vi "post_dust_event.vi"(8 "error in (no error)":errorcluster, 10 "Signal Array":T1[](array[typedef]), 11 "Cluster":T4 {"File Location" items=["Unknown"=-5, "IDL Processing"=-4, "Writing from Queue"=-3, "Labview Files"=-2, "Retry Labview files"=-1, "Local Cache "=0, "Storage"=1]}) -> (0 "error out":errorcluster, 1 "Experiment Settings":i32, 2 "Dust Event ID":i32, 3 "Test Server":bool)   [LabVIEW 2013]
uses:
  Public API/Post_Dust_Event.ctl
  Controls/File_location.ctl
  Public API/Signal.ctl
  Controls/Role ID.ctl
  Controls/Hardware ID.ctl
  <vilib>/addons/database/Auxilliary.llb/DB Tools Cursor Type.ctl
  <vilib>/addons/database/Connection.llb/Conn Execute.vi
  <vilib>/addons/database/Recordset.llb/Rec Fetch Recordset Data (R).vi
  <vilib>/addons/database/Recordset.llb/Rec Destroy - Connection.vi
  <vilib>/addons/database/_DB Variant To Data/Database Variant To Data.xnode
  <vilib>/addons/database/NI_Database_API.lvlib
panel:
  # "Signal"
  # "Dust Event"
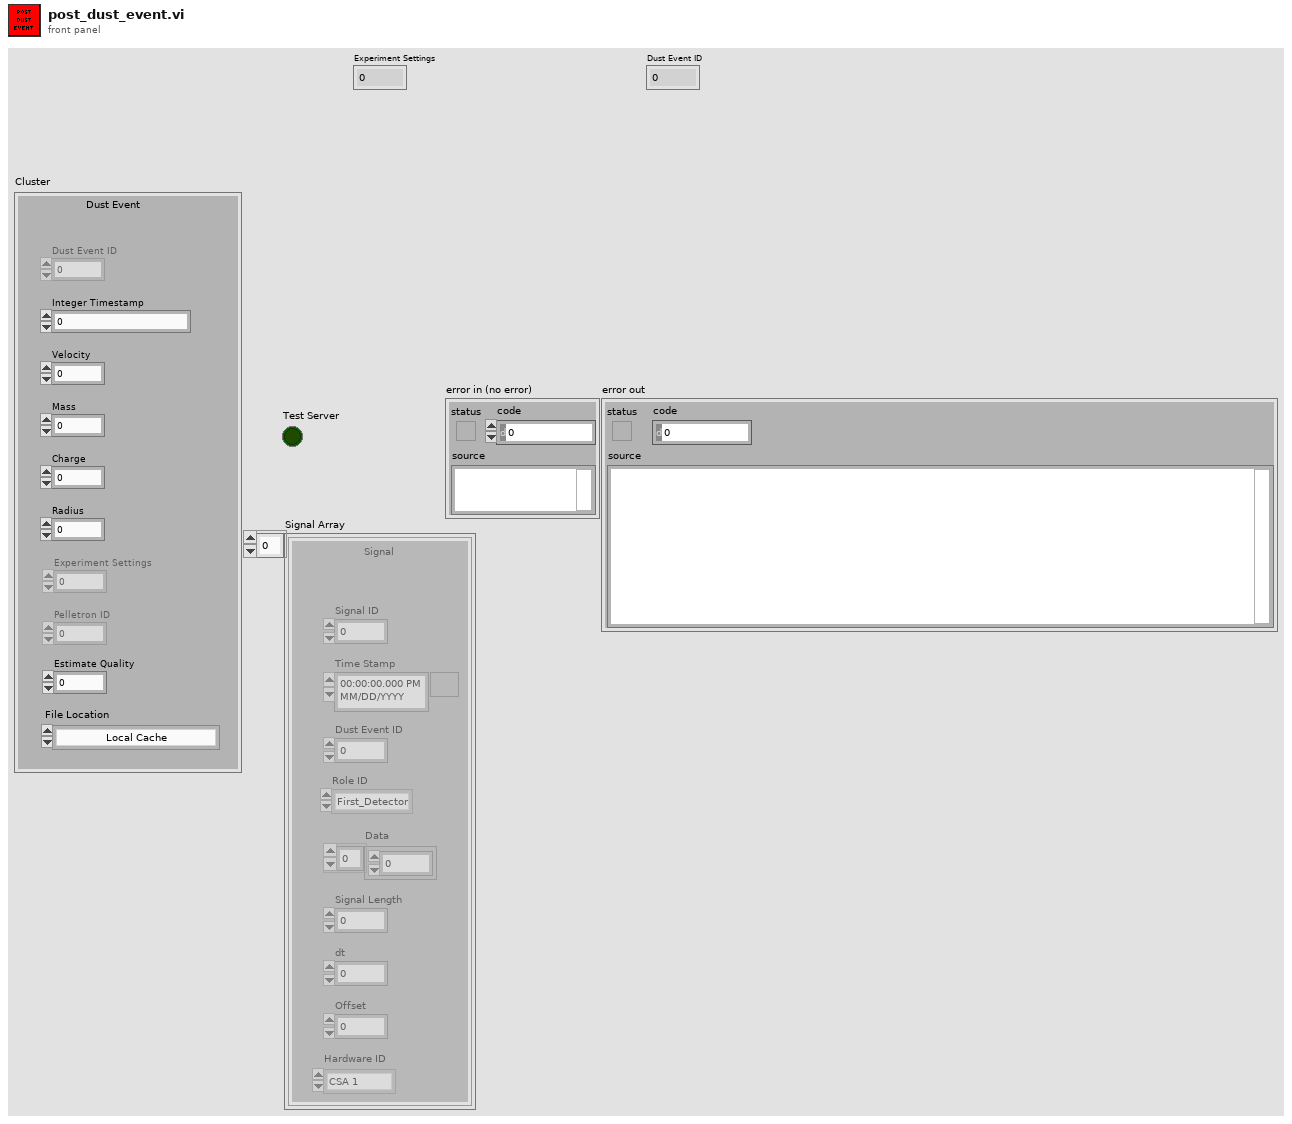
[diagram p1: front panel]
types:
  T1 = typedef "Signal.ctl" = cluster{"Signal ID":i64, "Time Stamp":timestamp, "Dust Event ID":i64, "Role ID":T2, "Data":sgl[], "Signal Length":i32, "dt":sgl, "Offset":dbl, "Hardware ID":T3}
  T2 = typedef "Role ID.ctl" = enum16{"First_Detector", "Second_Detector", "Third_Detector", "LeCroy_CH1", "LeCroy_CH2", "LeCroy_CH3", "LeCroy_CH4", "PSU"}
  T3 = typedef "Hardware ID.ctl" = enum16{"Unknown", "CSA 1", "CSA 2", "CSA 3", "CSA 4", "CSA 5", "CSA 6"}
  T4 = typedef "Post_Dust_Event.ctl" = cluster{"Dust Event ID":i64, "Integer Timestamp":i64, "Velocity":sgl, "Mass":sgl, "Charge":sgl, "Radius":sgl, "Experiment Settings":dbl, "Pelletron ID":i32, "Estimate Quality":sgl, "File Location":T5, "id_dust_info":dbl}
  T5 = typedef "File_location.ctl" = i8
  T6 = typedef "NI_Database_API.lvlib/DB Tools Cursor Type.ctl" = enum16{"forward-only", "keyset", "dynamic", "static"}
  T7 = typedef "NI_Database_API.lvlib/Conn ObjectReference.ctl" = refnum<k1>
  T8 = typedef "NI_Database_API.lvlib/Rec ObjectReference.ctl" = refnum<k1>
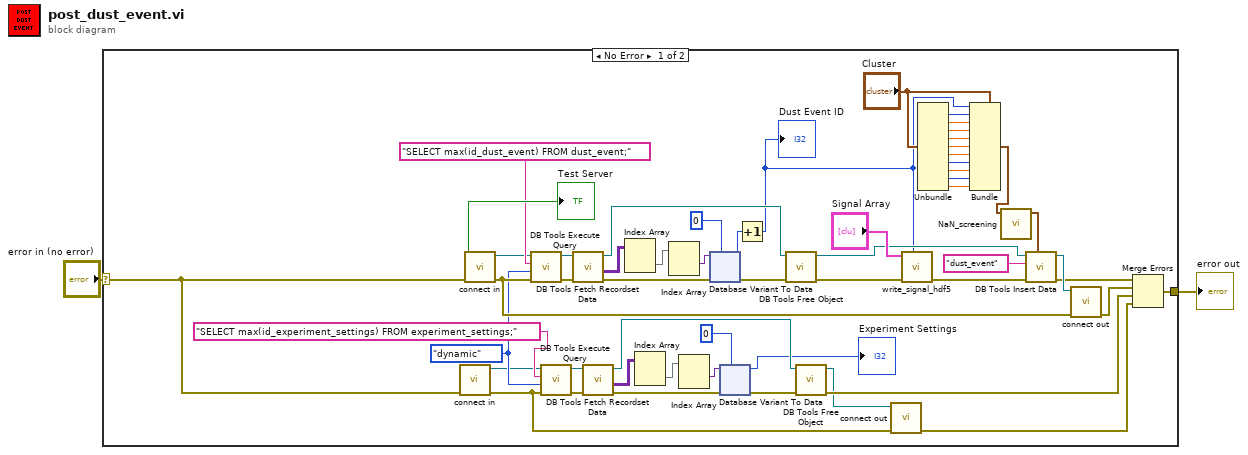
[diagram p0: block diagram]
diagram:
  n1 = case shown="No Error" "error in (no error)" {
    selector: "error in (no error)" -> [w7 w122]
    tunnel: [w56 w122] -> w1
    frame No Error {
      w11 = DB_Tools_Cursor_Type."dynamic" ("cursor type")
      n2 = call "connect in.vi"("error in (no error)"=w7) -> ("error out"=w4:errorcluster, "Database Connection"=w6:T7)  [unwired: 6 in, 1 out]
      n3 = call "connect in.vi"("error in (no error)"=w7) -> ("error out"=w13:errorcluster, "Database Connection"=w12:T7, "Test Server"=→"Test Server":bool)  [unwired: 6 in]
      n4 = call-poly <vilib>:"DB Tools Execute Query.vi"("error in (no error)"=w13, "cursor type"=w11, "SQL query"="SELECT max(id_dust_event) FROM dust_event;", "connection reference"=w12) -> ("error out"=w54:errorcluster, "recordset reference"=w55:T8)  [unwired: 4 in]
      n5 = call-poly <vilib>:"DB Tools Execute Query.vi"("error in (no error)"=w4, "cursor type"=w11, "SQL query"="SELECT max(id_experiment_settings) FROM experiment_settings;", "connection reference"=w6) -> ("error out"=w16:errorcluster, "recordset reference"=w15:T8)  [unwired: 4 in]
      n6 = call-poly <vilib>:"DB Tools Fetch Recordset Data.vi"("error in (no error)"=w54, "recordset reference"=w55) -> ("error out"=w49:errorcluster, "recordset data"=w51:variant[][], "recordset reference out"=w53:T8)  [unwired: 3 in]
      n7 = call-poly <vilib>:"DB Tools Fetch Recordset Data.vi"("error in (no error)"=w16, "recordset reference"=w15) -> ("error out"=w20:errorcluster, "recordset data"=w18:variant[][], "recordset reference out"=w17:T8)  [unwired: 3 in]
      n8 = Index Array(array=w51) -> (element=w42:variant[])  [unwired: 2 in]
      n9 = Index Array(array=w18) -> (element=w22:variant[])  [unwired: 2 in]
      n10 = Index Array(array=w42) -> (element #1=w43:variant)  [unwired: 2 in, 1 out]
      n11 = Index Array(array=w22) -> (element #1=w21:variant)  [unwired: 2 in, 1 out]
      n12 = xnode "Database Variant To Data"("database variant"=w43, "error in (no error)"=w49, "type"=0) -> ("data"=w44:i32, "error out"=w24:errorcluster)
      n13 = xnode "Database Variant To Data"("database variant"=w21, "error in (no error)"=w20, "type"=0) -> ("data"=→"Experiment Settings":i32, "error out"=w23:errorcluster)
      n14 = Increment(x=w44) -> (x+1=w26:i32)
      "Dust Event ID" <- w26
      n15 = call-poly <vilib>:"DB Tools Free Object.vi"("error in (no error)"=w24, "recordset reference"=w53) -> ("error out"=w45:errorcluster, "connection reference"=w40:T7)  [unwired: 8 in]
      n16 = call-poly <vilib>:"DB Tools Free Object.vi"("error in (no error)"=w23, "recordset reference"=w17) -> ("error out"=w8:errorcluster, "connection reference"=w5:T7)  [unwired: 8 in]
      n17 = call "connect out.vi"("error in (no error)"=w4, "connection reference"=w5) -> ("error out"=w3:errorcluster)  [unwired: 9 in]
      n18 = call "write_signal_hdf5.vi"("Index"=w26, "error in"=w45, "Signal array"="Signal Array") -> ("error out"=w41:errorcluster)  [unwired: 7 in, 1 out]
      n19 = Unbundle("Cluster") -> ("Integer Timestamp"=w27:i64, "Velocity"=w28:sgl, "Mass"=w29:sgl, "Charge"=w30:sgl, "Radius"=w31:sgl, "Experiment Settings"=w32:dbl, "Pelletron ID"=w33:i32, "Estimate Quality"=w34:sgl, "File Location"=w25:T5, "id_dust_info"=w35:dbl)  [unwired: 1 out]
      n20 = Bundle(cluster="Cluster", "Dust Event ID"=w26, "Integer Timestamp"=w27, "Velocity"=w28, "Mass"=w29, "Charge"=w30, "Radius"=w31, "Experiment Settings"=w32, "Pelletron ID"=w33, "Estimate Quality"=w34, "File Location"=w25, "id_dust_info"=w35) -> (w36:T4)
      n21 = call "NaN_screening.vi"("Input"=w36) -> ("Output"=w48:T4)  [unwired: 10 in]
      n22 = call <vilib>:"DB Tools Insert Data.vi"("data"=w48, "error in (no error)"=w41, "table"="dust_event", "connection reference"=w40) -> ("error out"=w38:errorcluster, "connection reference out"=w39:T7)  [unwired: 6 in]
      n23 = call "connect out.vi"("error in (no error)"=w13, "connection reference"=w39) -> ("error out"=w9:errorcluster)  [unwired: 9 in]
      n24 = Merge Errors(w38, w9, w8, w3) -> (w56:errorcluster)
    }
    frame Error {
    }
  }
  "error out" <- w1
